vi "PIDTuner.vi"() -> ()   [LabVIEW 2017]
uses:
  <vilib>/Rock Robotics/WPI/SafetyOutput/WPI_SafetyOutputConfigMenu.ctl
  <vilib>/Rock Robotics/SystemInterfaces/DIO/FPGA_DIOPWMChannel.ctl
  <vilib>/Rock Robotics/WPI/ThirdParty/Sensors/navX/_TypeDefs/FRIC_navX_DeviceNumbersTypeDef.ctl
  <vilib>/Rock Robotics/WPI/RobotDrive/WPI_RobotDriveOpen4MotorWithSPARK.vi
  <vilib>/Rock Robotics/WPI/RobotDrive/WPI_RobotDriveOpen2MotorWithSPARK.vi
  <vilib>/Rock Robotics/WPI/ThirdParty/Sensors/navX/_Processing Loop/FRIC_navX_Internal_SPI_ProcessingLoop.vi
panel:
  in  "Ouput":dbl(slide) scale=-1.0..1.0
  in  "ManualOverrride":bool
  in  "Disable Range":dbl=3.0
  in  "Integral Range":dbl=25.0
  in  "output range":cluster{"output high":dbl, "output low":dbl}={"output high"=0.65, "output low"=-0.65}
  out "Setpoint":cluster{"B":dbl, dbl}(graph)
  in  "A or B":bool=TRUE
  in  "B":dbl
  in  "A":dbl
  out "In Range":bool
  in  "Points":cluster{"X":dbl, "Y":dbl}[](array[cluster])=[{"X"=0.0, "Y"=0.0}, {"X"=0.01, "Y"=0.0}, {"X"=0.011, "Y"=0.3}, {"X"=1.0, "Y"=1.0}]
  in  "PID gains":T1={"proportional gain (Kc)"=0.003, "integral time (Ti, min)"=0.0, "derivative time (Td, min)"=0.0} {"derivative time (Td, min)" format="%#_9g"}
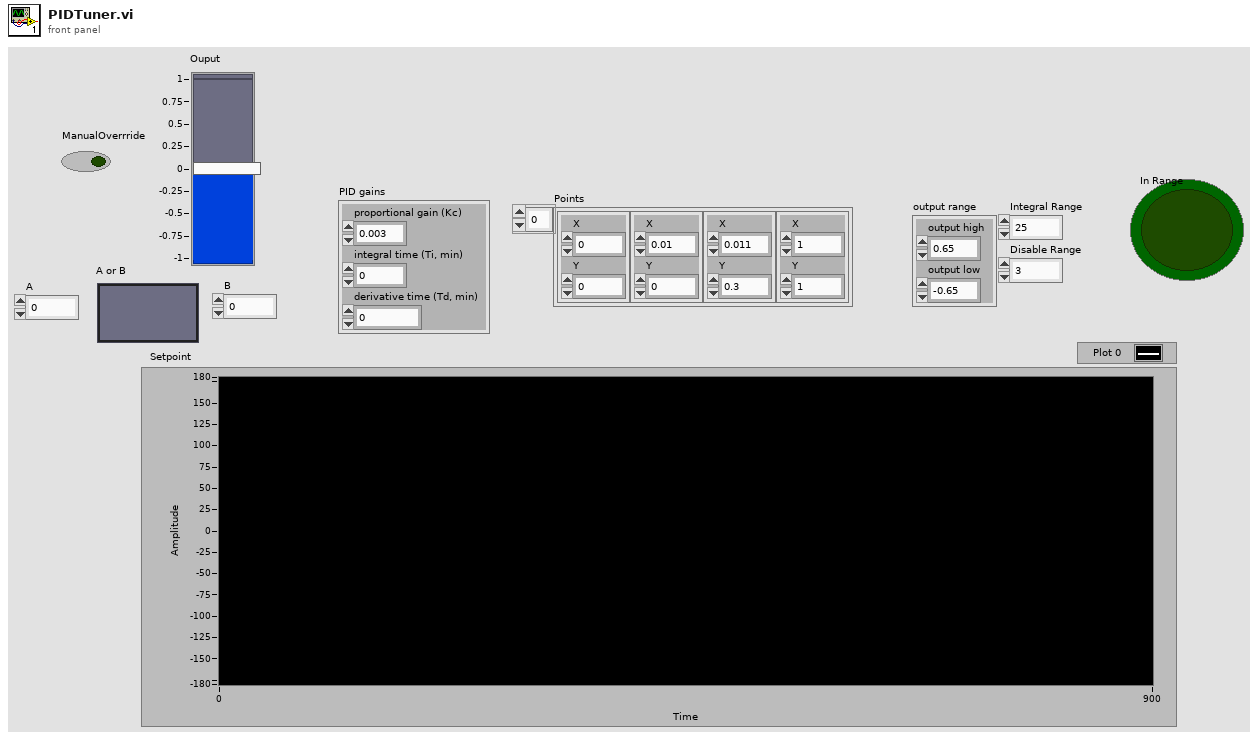
[diagram p1: front panel]
types:
  T1 = cluster{"proportional gain (Kc)":dbl, "integral time (Ti, min)":dbl, "derivative time (Td, min)":dbl}
  T2 = typedef "FRIC_navX_DeviceNumbersTypeDef.ctl" = enum16{"Dev0", "Dev1", "Dev2", "Dev3"}
  T3 = typedef "FPGA_DIOPWMChannel.ctl" = enum8{"PWM 0", "PWM 1", "PWM 2", "PWM 3", "PWM 4", "PWM 5", "PWM 6", "PWM 7", "PWM 8", "PWM 9", "PWM MXP 0", "PWM MXP 1", "PWM MXP 2", "PWM MXP 3", "PWM MXP 4", "PWM MXP 5", "PWM MXP 6", "PWM MXP 7", "PWM MXP 8", "PWM MXP 9", "Invalid"}
  T4 = typedef "WPI_SafetyOutputConfigMenu.ctl" = enum16{"Enable", "Disable"}
  T5 = typedef "WPI_RobotDriveDevRef.ctl" = cluster{"DevStatus":errorcluster, "Motors[]":T6[], "Square Inputs":bool, "Max Output":dbl}
  T6 = typedef "WPI_MotorControlDeviceRef.ctl" = cluster{"DeviceStatus":errorcluster, "Type":T7, "PWM":cluster{"PWM Channel":T3, "DeadBand":T8}, "CAN":cluster{"Device Number":u8, "SetOutput VI Ref":variant, "GetOutput VI Ref":variant, "Enable VI Ref":variant, "Disable VI Ref":variant, "Data":variant}, "Invert":bool, "DIO PWM":cluster{"PWM \"Enable\" Channel":T3, "DIOChannel":T9, "PWM Rate":dbl}}
  T7 = typedef "WPI_MotorControlType.ctl" = enum16{"PWM", "CAN", "DIO PWM"}
  T8 = typedef "WPI_PWMDeadband.ctl" = cluster{"Name":string, "maxPositivePwm":i32, "minPositivePwm":i32, "centerPwm":i32, "maxNegativePwm":i32, "minNegativePwm":i32, "angularRange":u16}
  T9 = typedef "FPGA_DIOChannel.ctl" = enum8{"DIO 0", "DIO 1", "DIO 2", "DIO 3", "DIO 4", "DIO 5", "DIO 6", "DIO 7", "DIO 8", "DIO 9", "DIO MXP 0", "DIO MXP 1", "DIO MXP 2", "DIO MXP 3", "DIO MXP 4", "DIO MXP 5", "DIO MXP 6", "DIO MXP 7", "DIO MXP 8", "DIO MXP 9", "DIO MXP 10", "DIO MXP 11", "DIO MXP 12", "DIO MXP 13", "DIO MXP 14", "DIO MXP 15", "SPI Port CS1", "SPI Port CS2", "SPI Port CS3", "SPI Port MISO", "SPI Port MOSI", "Invalid"}
  T10 = cluster{"Yaw":dbl, "Roll":dbl, "Pitch":dbl, "Heading":dbl, "Fused Heading":dbl}
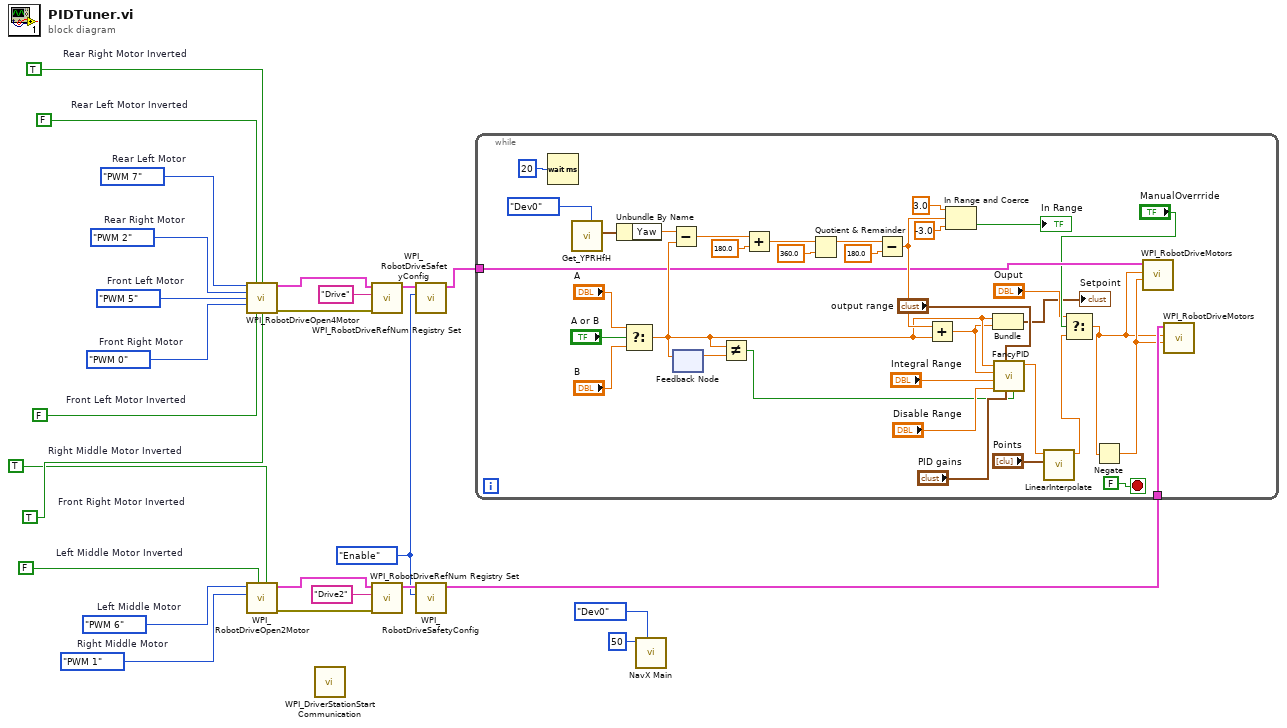
[diagram p0: block diagram]
diagram:
  w9 = TRUE  # Right Middle Motor Inverted
  w10 = FALSE  # Left Middle Motor Inverted
  w13 = FPGA_DIOPWMChannel."PWM 1"  # Right Middle Motor
  w14 = FPGA_DIOPWMChannel."PWM 6"  # Left Middle Motor
  w15 = TRUE  # Front Right Motor Inverted
  w16 = FALSE  # Front Left Motor Inverted
  w17 = TRUE  # Rear Right Motor Inverted
  w18 = FALSE  # Rear Left Motor Inverted
  w19 = FPGA_DIOPWMChannel."PWM 0"  # Front Right Motor
  w20 = FPGA_DIOPWMChannel."PWM 5"  # Front Left Motor
  w21 = FPGA_DIOPWMChannel."PWM 2"  # Rear Right Motor
  w22 = FPGA_DIOPWMChannel."PWM 7"  # Rear Left Motor
  w5 = WPI_SafetyOutputConfigMenu."Enable" ("mode")
  n1 = call-poly <vilib>:"WPI_RobotDriveOpen4Motor.vi"("Rear Left Motor"=w22, "Rear Left Motor Inverted"=w18, "Rear Right Motor Inverted"=w17, "Rear Right Motor"=w21, "Front Left Motor"=w20, "Front Right Motor"=w19, "Front Left Motor Inverted"=w16, "Front Right Motor Inverted"=w15) -> ("RobotDriveDevRef"=w25:T5, "error out"=w23:errorcluster)  [unwired: 6 in]
  n2 = call-poly <vilib>:"WPI_RobotDriveOpen2Motor.vi"("Right Motor Inverted"=w9, "Left Motor Inverted"=w10, "Right Motor"=w13, "Left Motor"=w14) -> ("error out"=w8:errorcluster, "RobotDriveDevRef"=w12:T5)  [unwired: 6 in]
  n3 = call <vilib>:"WPI_DriverStationStart Communication.vi"() -> ()  [unwired: 12 in]
  n4 = call <vilib>:"WPI_RobotDriveRefNum Registry Set.vi"("error in (no error)"=w23, "refnum name"="Drive", "RobotDriveDevRef"=w25) -> ("RobotDriveDevRef"=w7:T5)  [unwired: 1 in, 7 out]
  n5 = call <vilib>:"WPI_RobotDriveRefNum Registry Set.vi"("error in (no error)"=w8, "refnum name"="Drive2", "RobotDriveDevRef"=w12) -> ("RobotDriveDevRef"=w6:T5)  [unwired: 7 in, 1 out]
  n6 = call <vilib>:"WPI_RobotDriveSafetyConfig.vi"("mode"=w5, "RobotDriveDevRef"=w7) -> ("RobotDriveDevRef"=w4:T5)  [unwired: 8 in, 1 out]
  n7 = call <vilib>:"WPI_RobotDriveSafetyConfig.vi"("mode"=w5, "RobotDriveDevRef"=w6) -> ("RobotDriveDevRef"=w3:T5)  [unwired: 8 in, 1 out]
  n8 = while {
    tunnel: w4 -> [w33]
    tunnel: w3 -> [w32]
    stop <- FALSE stop-if-true
    n9 = Wait (ms)(milliseconds to wait=u32 20) -> ()  [unwired: 1 out]
    n10 = call <vilib>:"Get_YPRHfH.vi"("Device Number"=FRIC_navX_DeviceNumbersTypeDef."Dev0") -> ("YRPHfH"=w57:T10)  [unwired: 10 in]
    n11 = Unbundle By Name(w57) -> ("Yaw"=w49:dbl)
    n12 = Select(t="A", s="A or B", f="B") -> (s? t:f=w40:dbl)
    n13 = Subtract(x=w49, y=w40) -> (x-y=w50:dbl)
    n14 = feedback-in #1(w40) -> ()
    n15 = feedback #1() -> (w42:dbl)  [unwired: 1 in]
    n16 = Not Equal?(x=w40, y=w42) -> (x != y?=w34:bool)
    n17 = Add(x=w50, y=180.0) -> (x+y=w53:dbl)
    n18 = Quotient & Remainder(x=w53, y=360.0) -> (x-y*floor(x/y)=w51:dbl)  [unwired: 1 out]
    n19 = Subtract(x=w51, y=180.0) -> (x-y=w43:dbl)
    n20 = Add(x=w43, y=w40) -> (x+y=w39:dbl)
    n21 = In Range and Coerce(upper limit=3.0, x=w43, lower limit=-3.0) -> (In Range?=→"In Range":bool)  [unwired: 1 out]
    n22 = Bundle("B"=w40, w39) -> (→"Setpoint":cluster{"B":dbl, dbl})  [unwired: 1 in]
    n23 = call "FancyPID.vi"("Reset"=w34, "Gains"="PID gains", "Range"="output range", "Disable Range"="Disable Range", "Integral Range"="Integral Range", "Process variable"=w39, "Setpoint"=w40) -> ("output"=w36:dbl)  [unwired: 4 in]
    n24 = call "LinearInterpolate.vi"("Points"="Points", "Value"=w36) -> ("Output"=w30:dbl)  [unwired: 9 in]
    n25 = Select(t="Ouput", s="ManualOverrride", f=w30) -> (s? t:f=w28:dbl)
    n26 = Negate(x=w28) -> (-x=w31:dbl)
    n27 = call <vilib>:"WPI_RobotDriveMotors.vi"("RightSpeed"=w31, "LeftSpeed"=w28, "RobotDriveDevRef"=w33) -> ()  [unwired: 1 in, 8 out]
    n28 = call <vilib>:"WPI_RobotDriveMotors.vi"("RightSpeed"=w31, "LeftSpeed"=w28, "RobotDriveDevRef"=w32) -> ()  [unwired: 1 in, 8 out]
  }
  n29 = call-poly <vilib>:"NavX Main.vi"("Device Number"=FRIC_navX_DeviceNumbersTypeDef."Dev0", "Rate (4Hz-200Hz)"=u8 50) -> ()  [unwired: 10 in]
